vi "Get Device Info.vi"(8 "error in (no error)":errorcluster) -> (0 "error out":errorcluster, 1 "Is Running":bool[](array[boolean]), 2 "Kinect Properties":T1(array[cluster]), 3 "Number of Kinects Attached":i32)   [LabVIEW 2014, in "Kinect Library.lvlib"]
doc: "This VI returns an array of information about all Kinect sensors attached to this computer. This information can be used to decide which Kinect to interface with using the Initialize Kinect VI."
uses:
  Kinect Library.lvlib
  Microsoft.Kinect
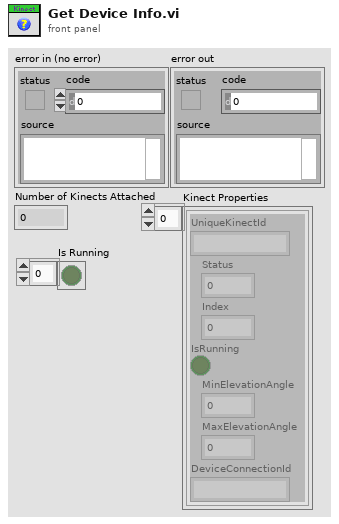
[diagram p1: front panel]
types:
  T1 = cluster{"UniqueKinectId":string, "Status":i32, "Index":i32, "IsRunning":bool, "MinElevationAngle":i32, "MaxElevationAngle":i32, "DeviceConnectionId":string}[]
  T2 = cluster{"UniqueKinectId":string, "Status":i32, "Index":i32, "IsRunning":bool, "MinElevationAngle":i32, "MaxElevationAngle":i32, "DeviceConnectionId":string}
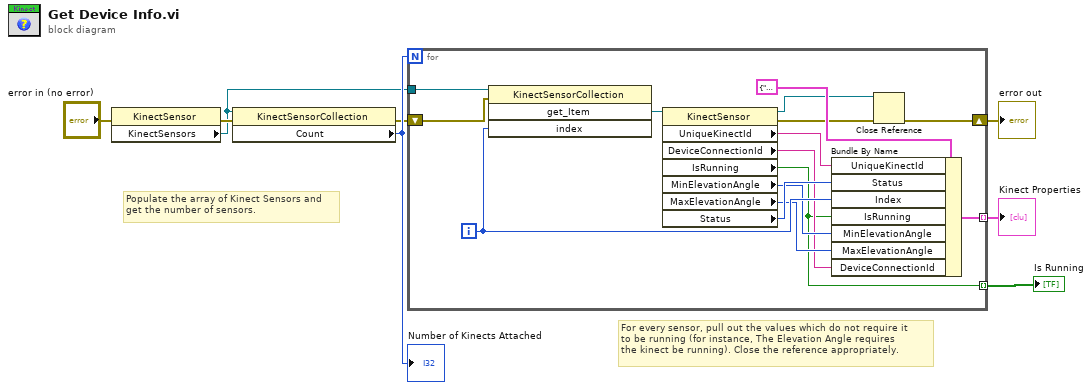
[diagram p0: block diagram]
diagram:
  # "For every sensor, pull out the values which do not require it\nto be running (for instance, The Elevation Angle requires\nthe kinect be running). Close the reference appropriately."
  # "Populate the array of Kinect Sensors and\nget the number of sensors."
  n1 = property class="KinectSensor"(error in="error in (no error)") -> (error out=w7:errorcluster, "KinectSensors"=w5:refnum<k24>)  [unwired: 1 in, 1 out]
  n2 = property class="KinectSensorCollection"(reference=w5, error in=w7) -> (error out=w4:errorcluster, "Count"=w6:i32)  [unwired: 1 out]
  "Number of Kinects Attached" <- w6
  n3 = for {
    N: w6 -> [_]
    tunnel: w5 -> [w23]
    tunnel: [w16] -> w2 mode=indexing
    shift-right: [w12] -> w3
    shift-left: w4 -> [w15]
    tunnel: [w9] -> w1 mode=indexing
    i -> [w21]
    n4 = invoke class="KinectSensorCollection" method="get_Item"(reference=w23, error in=w15, "index"=w21) -> ("get_Item"=w11:refnum<k24>)  [unwired: 1 in, 3 out]
    n5 = property class="KinectSensor"(reference=w11) -> (reference out=w13:refnum<k24>, error out=w14:errorcluster, "UniqueKinectId"=w20:string, "DeviceConnectionId"=w10:string, "IsRunning"=w9:bool, "MinElevationAngle"=w18:i32, "MaxElevationAngle"=w17:i32, "Status"=w19:i32)  [unwired: 1 in]
    n6 = Bundle By Name(cluster=T2 {"UniqueKinectId"="", "Status"=0, "Index"=0, "IsRunning"=FALSE, "MinElevationAngle"=0, "MaxElevationAngle"=0, "DeviceConnectionId"=""}, "UniqueKinectId"=w20, "Status"=w19, "Index"=w21, "IsRunning"=w9, "MinElevationAngle"=w18, "MaxElevationAngle"=w17, "DeviceConnectionId"=w10) -> (w16:T2)
    n7 = Close Reference(reference=w13, error in (no error)=w14) -> (error out=w12:errorcluster)
  }
  "error out" <- w3
  "Kinect Properties" <- w2
  "Is Running" <- w1
